vi "Configure Linear Step Mode Sweep.vi"(0 "VISA resource name":refnum<visa-resource-name>, 1 "Source Mode  (0: Voltage)":u16(ring) items=["Voltage", "Current"], 2 "Sweep Points":cluster{"Start ":dbl, "Stop ":dbl, "Step":dbl}={"Start "=0.0, "Stop "=1.0, "Step"=0.1}, 3 "Delay (-1)":dbl=-1.0, 4 "Count (1)":i32=1, 5 "error in (no error)":errorcluster, 6 "Fail Abort (T:ON)":bool=TRUE, 7 "Range Type  (1: Best Fixed Range)":u16(ring)=1 items=["Most Sensitive Source Range", "Best Fixed Range", "Present Source Range"], 8 "Dual (F:OFF)":bool, 9 "Buffer Name (defbuffer1)":string="defbuffer1") -> (14 "VISA resource name out":refnum<visa-resource-name>, 19 "error out":errorcluster)   [LabVIEW 2020, in "Keithley 2450.lvlib"]
doc: "Sets up a linear source sweep configuration list and trigger model with a fixed number of steps."
uses:
  Keithley 2450.lvlib
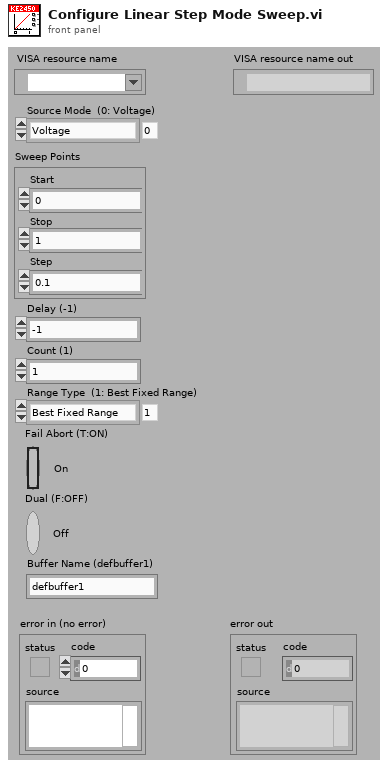
[diagram p1: front panel]
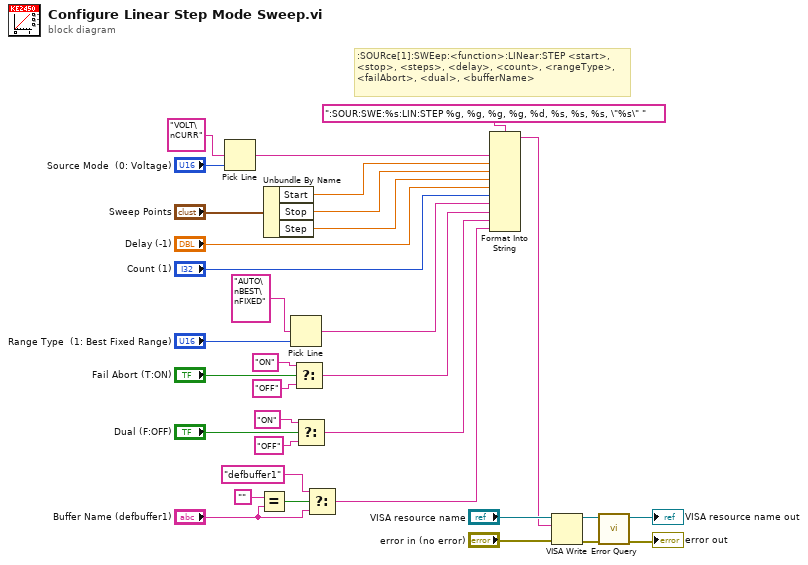
[diagram p0: block diagram]
diagram:
  # ":SOURce[1]:SWEep:<function>:LINear:STEP <start>, <stop>, <steps>, <delay>, <count>, <rangeType>, <failAbort>, <dual>, <bufferName>"
  n1 = Pick Line(multi-line string="VOLT\nCURR" ("string (\"\")"), line index="Source Mode  (0: Voltage)") -> (output string=w30:string)  [unwired: 1 out]
  n2 = Equal?(x="", y="Buffer Name (defbuffer1)") -> (x = y?=w7:bool)
  n3 = Unbundle By Name("Sweep Points") -> ("Start"=w22:dbl, "Stop"=w21:dbl, "Step"=w20:dbl)
  n4 = Pick Line(multi-line string="AUTO\nBEST\nFIXED" ("string (\"\")"), line index="Range Type  (1: Best Fixed Range)") -> (output string=w1:string)  [unwired: 1 out]
  n5 = Select(t="ON" ("Buffer Name (defbuffer1)"), s="Fail Abort (T:ON)", f="OFF" ("Buffer Name (defbuffer1)")) -> (s? t:f=w15:string)
  n6 = Select(t="ON" ("Buffer Name (defbuffer1)"), s="Dual (F:OFF)", f="OFF" ("Buffer Name (defbuffer1)")) -> (s? t:f=w9:string)
  n7 = Select(t="defbuffer1", s=w7, f="Buffer Name (defbuffer1)") -> (s? t:f=w5:string)
  n8 = Format Into String(format string=":SOUR:SWE:%s:LIN:STEP %g, %g, %g, %g, %d, %s, %s, %s, \"%s\" ", w30, w22, w21, w20, "Delay (-1)", "Count (1)", w1, w15, w9, w5) -> (resulting string=w16:string)  [unwired: 2 in, 1 out]
  n9 = VISA Write(VISA resource name="VISA resource name", write buffer=w16, error in (no error)="error in (no error)") -> (VISA resource name out=w27:refnum<visa-resource-name>, error out=w26:errorcluster)  [unwired: 1 out]
  n10 = call "Error Query.vi"("error in (no error)"=w26, "VISA resource name"=w27) -> ("error out"=→"error out":errorcluster, "VISA resource name out"=→"VISA resource name out":refnum<visa-resource-name>)  [unwired: 8 out]
